vi "Digital Blinking LED.vi"   [LabVIEW 2014]
doc: "This example shows how to set an Wemos D1 ESP8299 digital pin to an output, then toggle the voltage between low (0V) and high (3.3V) to drive an LED on and off."
uses:
  <vilib>/Aledyne-TSXperts/Arduino Compatible Compiler for LabVIEW/Code Generator/Arduino APIs/Digital/PinDirection.ctl
  <vilib>/Aledyne-TSXperts/Arduino Compatible Compiler for LabVIEW/Arduino Compatible Compiler for LabVIEW.lvlib
panel:
  # "Onboard LED: D5/D13/SCK"
types:
  T1 = typedef "Arduino Compatible Compiler for LabVIEW.lvlib/PinDirection.ctl" = enum16{" INPUT", "OUTPUT", " INPUT_PULLUP"}
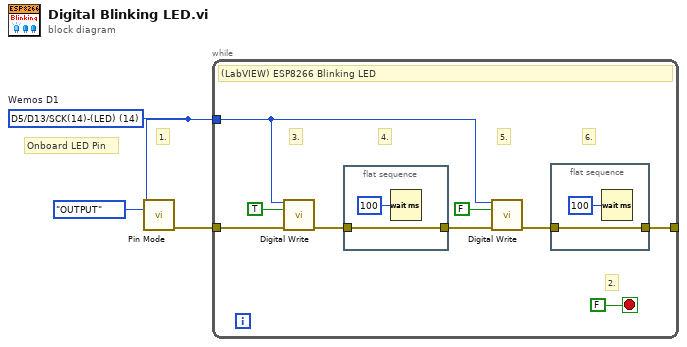
[diagram p0: block diagram]
diagram:
  w1 = u8 14 items=["D0-RX(3)"=3, "D1-TX(1)"=1, "D2(16)"=16, "D3/D15/SCL(5)"=5, "D4/D14/SDA(4)"=4, "D5/D13/SCK(14)-(LED)"=14, "D6/D12/MISO(12)"=12, "D7/D11/MOSI(13)"=13, "D8(0)"=0, "D9/TX1(2)"=2, "D10/SS (15)"=15, "ADC0,(17)"=17]  # Wemos D1
  # "Onboard LED Pin"
  # "1."
  n1 = call <vilib>:"Pin Mode.vi"("pin"=w1, "direction"=PinDirection."OUTPUT" ("Direction")) -> ("error out"=w3:errorcluster)  [unwired: 13 in]
  n2 = while {
    tunnel: w1 -> [w9]
    tunnel: w3 -> [w8]
    tunnel: [w10] -> _
    stop <- FALSE stop-if-true
    # "2."
    # "6."
    # "5."
    # "4."
    # "3."
    # "(LabVIEW) ESP8266 Blinking LED"
    n3 = call <vilib>:"Digital Write.vi"("pin"=w9, "state"=TRUE, "error in (no error)"=w8) -> ("error out"=w12:errorcluster)  [unwired: 12 in]
    n4 = flat-sequence {
      tunnel: [w15] -> w7
      tunnel: w12 -> [w15]
      frame #0 {
        n5 = Wait (ms)(milliseconds to wait=u32 100) -> ()  [unwired: 1 out]
      }
    }
    n6 = call <vilib>:"Digital Write.vi"("pin"=w9, "state"=FALSE, "error in (no error)"=w7) -> ("error out"=w11:errorcluster)  [unwired: 12 in]
    n7 = flat-sequence {
      tunnel: [w14] -> w10
      tunnel: w11 -> [w14]
      frame #0 {
        n8 = Wait (ms)(milliseconds to wait=u32 100) -> ()  [unwired: 1 out]
      }
    }
  }
